vi "simple magnet sweep (wait).vi"(10 "Set Rate":dbl[](array[numeric])=[0.1, 0.1, 0.1, 0.02, 0.02, 0.02, 0.01, 0.01], 11 "appended array":dbl[][](array[numeric])=[[0.0, 0.0, 9.0], [0.0, 0.0, -9.0], [0.0, 0.0, 0.0], [2.0, 0.0, 0.0], [-2.0, 0.0, 0.0], [0.0, 0.0, 0.0], [0.0, 2.0, 0.0], [0.0, -2.0, 0.0]]) -> ()   [LabVIEW 2013]
panel:
  in  "milliseconds to wait":u32=3600000
  out "temp":dbl=3693.7589267269373
  # "z: 0.1\nx: 0.02\ny: 0.01 T/min"
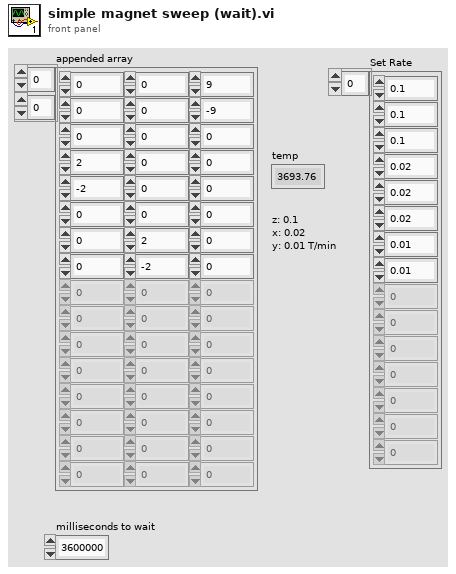
[diagram p1: front panel]
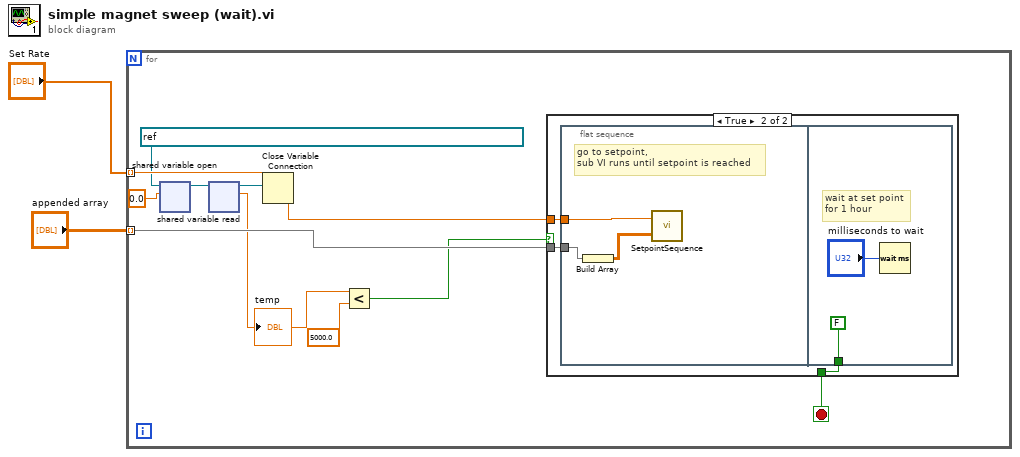
[diagram p0: block diagram]
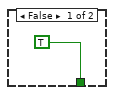
[diagram p2: hidden frame]
diagram:
  n1 = for {
    tunnel: "Set Rate" -> [w12] mode=indexing
    tunnel: "appended array" -> [w11] mode=indexing
    stop <- w4 stop-if-true
    n2 = shared-variable-open(refnum<k21> "ni.var.psp://housesoftheholy/Leiden CF900/Leiden CF TC/CF TC T0" ("shared variable refnum in"), 0.0) -> (w10:refnum<k21>)  [unwired: 2 in, 1 out]
    n3 = shared-variable-read(w10) -> (w9:refnum<k21>, w7:dbl)  [unwired: 1 in, 2 out]
    "temp" <- w7
    n4 = Close Variable Connection(11:w9) -> ()  [unwired: 1 in, 1 out]
    n5 = Less?(x=w7, y=5000.0) -> (x < y?=w6:bool)
    n6 = case shown="True" w6 {
      tunnel: w12 -> [_ w16]
      tunnel: w11 -> [_ w15]
      tunnel: [TRUE w14] -> w4
      frame False {
      }
      frame True {
        n7 = flat-sequence {
          tunnel: w16 -> [w19]
          tunnel: w15 -> [w18]
          tunnel: [FALSE] -> w14
          frame #0 {
            # "go to setpoint, \nsub VI runs until setpoint is reached"
            n8 = Build Array(w18) -> (w17:dbl[][])
            n9 = call "SetpointSequence.vi"("appended array"=w17, "Sweep rate (T/min)"=w19) -> ()  [unwired: 1 in, 1 out]
          }
          frame #1 {
            # "wait at set point\nfor 1 hour"
            n10 = Wait (ms)(milliseconds to wait="milliseconds to wait") -> ()  [unwired: 1 out]
          }
        }
      }
    }
  }
